vi "Update Control Labels.vi"(8 "error in":errorcluster, 10 "rename data":T3, 11 "vi reference in":refnum<vi>) -> (0 "error out":errorcluster, 2 "rename labels result":T1[](array[typedef]), 3 "vi reference out":refnum<vi>)   [LabVIEW 2021, in "MeasurementService Editor.lvlib"]
uses:
  MeasurementService Editor.lvlib
  RenameRefactor/Rename Refactor Data.ctl
  RenameRefactor/Rename Refactor Mapping Info.ctl
  RenameRefactor/Rename String Mapping.ctl
  RenameRefactor/Rename String Result.ctl
  RenameRefactor/Rename String.ctl
  5da6465f-a298-4a47-946a-c2e194c03798.vi
  <vilib>/Comparison/Equal/Equal Functor/Equal Functor.lvclass
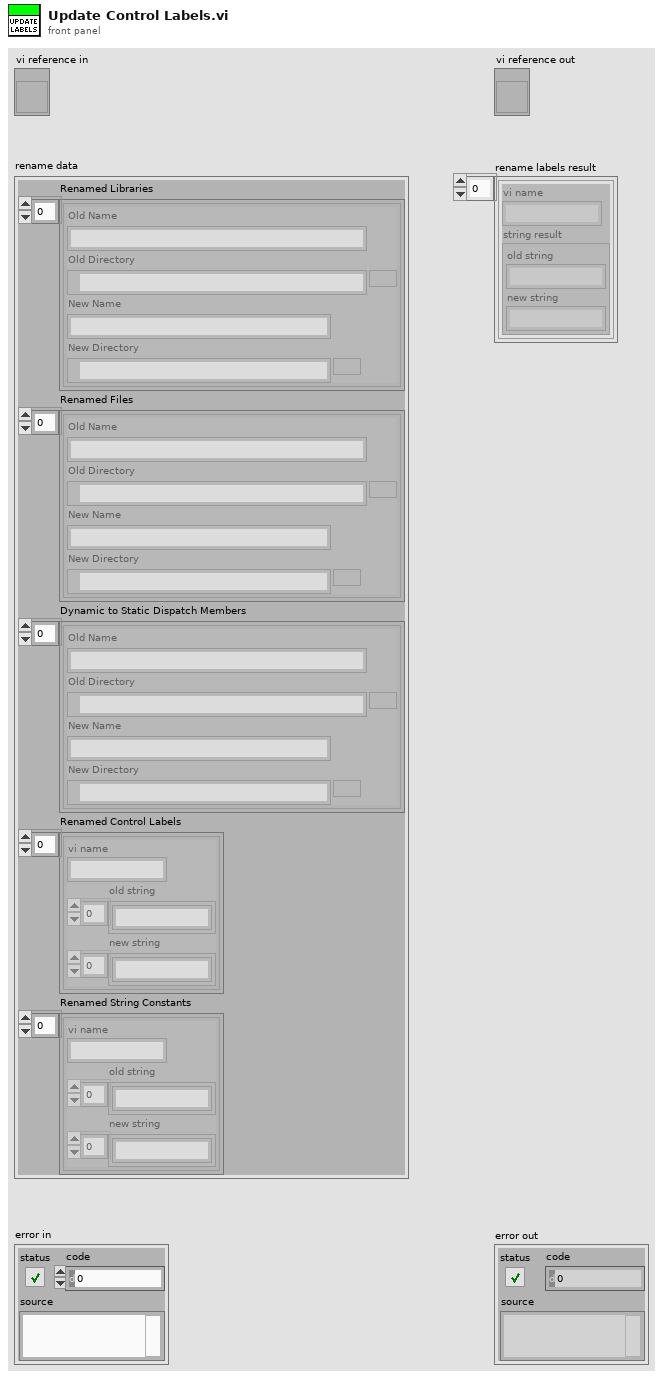
[diagram p1: front panel]
types:
  T1 = typedef "MeasurementService Editor.lvlib/Rename String Result.ctl" = cluster{"vi name":string, "string result":T2}
  T2 = typedef "MeasurementService Editor.lvlib/Rename String.ctl" = cluster{"old string":string, "new string":string}
  T3 = typedef "MeasurementService Editor.lvlib/Rename Refactor Data.ctl" = cluster{"Renamed Libraries":T4[], "Renamed Files":T4[], "Dynamic to Static Dispatch Members":T4[], "Renamed Control Labels":T5[], "Renamed String Constants":T5[]}
  T4 = typedef "MeasurementService Editor.lvlib/Rename Refactor Mapping Info.ctl" = cluster{"Old Name":string, "Old Directory":path, "New Name":string, "New Directory":path}
  T5 = typedef "MeasurementService Editor.lvlib/Rename String Mapping.ctl" = cluster{"vi name":string, "old string":string[], "new string":string[]}
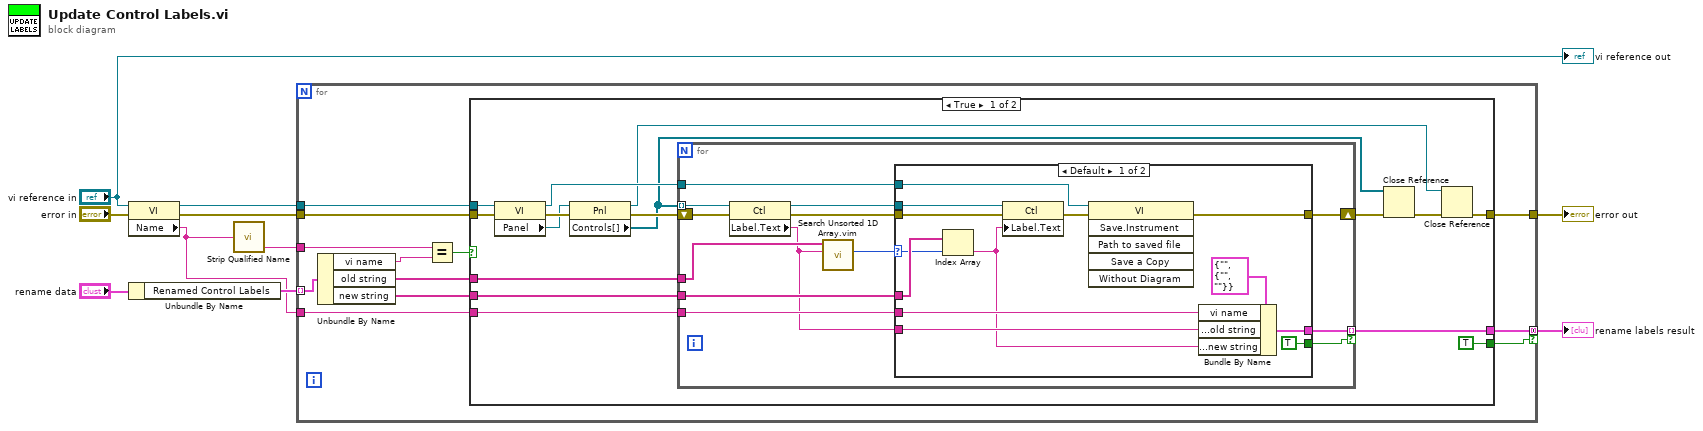
[diagram p0: block diagram]
diagram:
  n1 = property class="VI"(reference="vi reference in", error in="error in") -> (reference out=w6:refnum<vi>, error out=w8:errorcluster, "Name"=w2:string)
  n2 = Unbundle By Name("rename data") -> ("Renamed Control Labels"=w4:T5[])
  n3 = call "Strip Qualified Name.vi"("name"=w2) -> ("last name"=w9:string)  [unwired: 5 in, 1 out]
  n4 = for {
    tunnel: w9 -> [w22]
    tunnel: w4 -> [w21] mode=indexing
    tunnel: w6 -> [w18]
    tunnel: w8 -> [w17]
    tunnel: [w16] -> w7
    tunnel: w2 -> [w13]
    tunnel: [w12] -> w1 mode=concatenating if=w11
    n5 = Unbundle By Name(w21) -> ("vi name"=w20:string, "old string"=w15:string[], "new string"=w14:string[])
    n6 = Equal?(x=w22, y=w20) -> (x = y?=w19:bool)
    n7 = case shown="True" w19 {
      tunnel: w18 -> [w35 _]
      tunnel: w17 -> [w36 w66]
      tunnel: [w30 w66] -> w16
      tunnel: w15 -> [w38 _]
      tunnel: w14 -> [w37 _]
      tunnel: w13 -> [w25 _]
      tunnel: [w24 _] -> w12
      tunnel: [TRUE _] -> w11
      frame True {
        n8 = property class="VI"(reference=w35, error in=w36) -> (reference out=w32:refnum<vi>, error out=w34:errorcluster, "Panel"=w33:refnum<vi>)
        n9 = property class="Pnl"(reference=w33, error in=w34) -> (reference out=w29:refnum<vi>, error out=w31:errorcluster, "Controls[]"=w26:refnum<vi>[])
        n10 = for {
          tunnel: w26 -> [w50] mode=indexing
          shift-right: [w49] -> w28
          shift-left: w31 -> [w51]
          tunnel: w38 -> [w46]
          tunnel: w37 -> [w44]
          tunnel: w32 -> [w43]
          tunnel: w25 -> [w42]
          tunnel: [w40] -> w24 mode=indexing if=w39
          n11 = property class="Ctl"(reference=w50, error in=w51) -> (reference out=w48:refnum<vi>, error out=w47:errorcluster, "Label.Text"=w41:string)
          n12 = call "Search Unsorted 1D Array.vim"("element"=w41, "unsorted 1D array"=w46) -> ("index of element"=w45:i32)  [unwired: 9 in]
          n13 = case shown="Default" w45 {
            selector: w45 -> [w61 _]
            tunnel: [w58 w65] -> w49
            tunnel: w48 -> [w64 _]
            tunnel: w47 -> [w63 w65]
            tunnel: w44 -> [w62 _]
            tunnel: w43 -> [w59 _]
            tunnel: w42 -> [w56 _]
            tunnel: w41 -> [w55 _]
            tunnel: [w53 _] -> w40
            tunnel: [TRUE _] -> w39
            frame Default {
              n14 = Index Array(array=w62, index=w61) -> (element=w54:string)
              n15 = property class="Ctl"(reference=w64, error in=w63, "Label.Text"=w54) -> (error out=w60:errorcluster)  [unwired: 1 out]
              n16 = invoke class="VI" method="Save.Instrument"(reference=w59, error in=w60) -> (error out=w58:errorcluster)  [unwired: 4 in, 5 out]
              n17 = Bundle By Name(cluster=T1 {"vi name"="", "string result"={"old string"="", "new string"=""}}, "vi name"=w56, "string result.old string"=w55, "string result.new string"=w54) -> (w53:T1)
            }
            frame -1 {
            }
          }
        }
        n18 = Close Reference(reference=w26, error in (no error)=w28) -> (error out=w27:errorcluster)
        n19 = Close Reference(reference=w29, error in (no error)=w27) -> (error out=w30:errorcluster)
      }
      frame False {
      }
    }
  }
  "error out" <- w7
  "rename labels result" <- w1
  "vi reference out" <- "vi reference in"
